vi "DriveControl.vi"(5 "RobotDriveDevRef":T1={"DevStatus"={"status"=FALSE, "code"=0, "source"=""}, "Motors[]"=[], "Square Inputs"=FALSE, "Max Output"=1.0, "Isochronous"=FALSE}, 7 "Xvalue of Target":dbl, 8 "Right axis value":dbl, 9 "Left axis value":dbl, 10 "Lower Bound":dbl, 11 "Upper Bound":dbl) -> (1 "Set Right Speed":dbl, 2 "Set Left Speed":dbl, 3 "RobotDriveDevRef":T1={"DevStatus"={"status"=FALSE, "code"=0, "source"=""}, "Motors[]"=[], "Square Inputs"=FALSE, "Max Output"=1.0, "Isochronous"=FALSE})   [LabVIEW 2011]
uses:
  <vilib>/Rock Robotics/WPI/RobotDrive/WPI_RobotDriveDevRef.ctl
  <vilib>/Rock Robotics/WPI/MotorControl/WPI_MotorControlDeviceRef.ctl
  <vilib>/Rock Robotics/SystemInterfaces/Typedef/FPGA_TypedefDigitalModule.ctl
  <vilib>/Rock Robotics/SystemInterfaces/DIO/FPGA_DIOPWMChannel.ctl
  <vilib>/Rock Robotics/WPI/PWM/WPI_PWMDeadband.ctl
  <vilib>/Rock Robotics/WPI/CAN/Jaguar/SubVIs/WPI_CANJaguar_ControlMode.ctl
  <vilib>/Rock Robotics/WPI/PWM/WPI_PWMTransform_ConPane.ctl
  System Set Points and States.vi
panel:
  in  "Joystick value":dbl
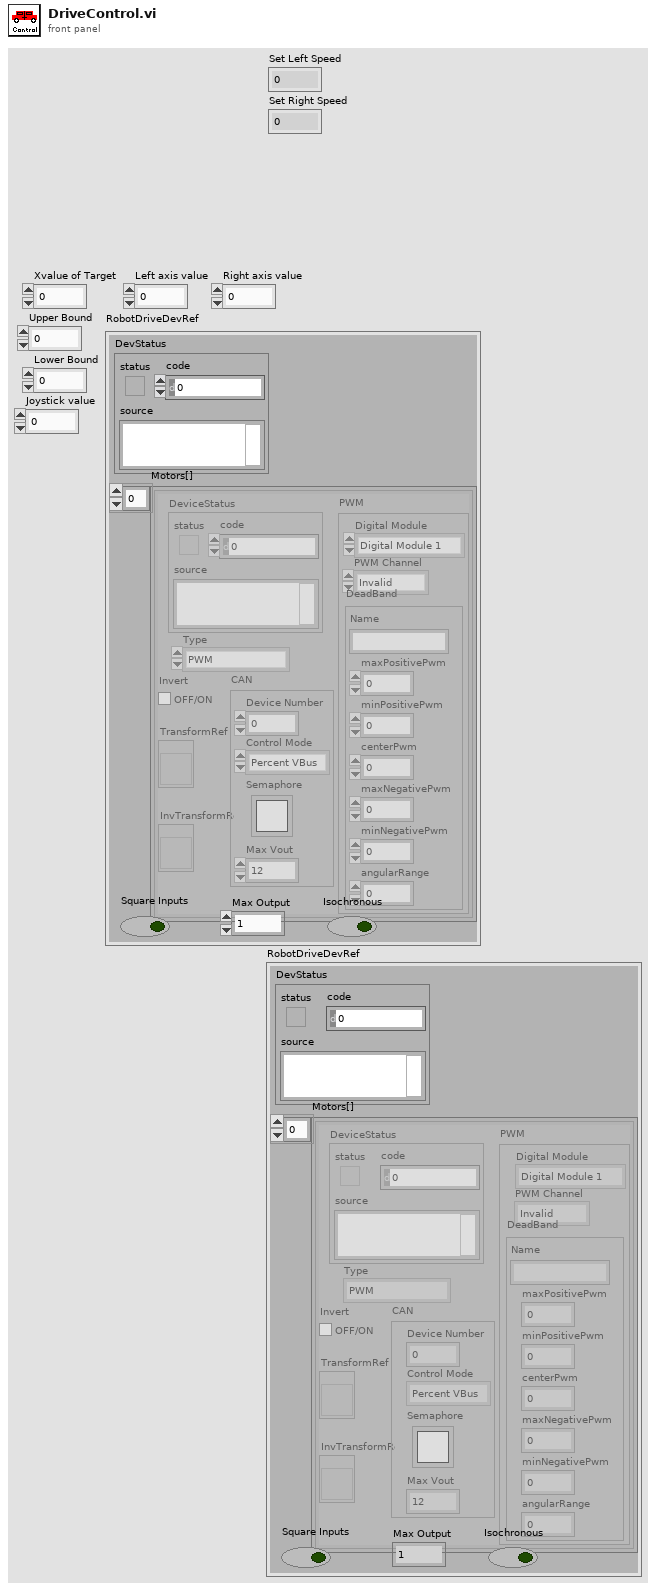
[diagram p1: front panel]
types:
  T1 = typedef "WPI_RobotDriveDevRef.ctl" = cluster{"DevStatus":errorcluster, "Motors[]":T2[], "Square Inputs":bool, "Max Output":dbl, "Isochronous":bool}
  T2 = typedef "WPI_MotorControlDeviceRef.ctl" = cluster{"DeviceStatus":errorcluster, "Type":enum16{"PWM", "CAN"}, "PWM":cluster{"Digital Module":T3, "PWM Channel":T4, "DeadBand":T5}, "CAN":cluster{"Device Number":u8, "Control Mode":T6, "Semaphore":T7, "Max Vout":dbl}, "Invert":bool, "TransformRef":T8, "InvTransformRef":T8}
  T3 = typedef "FPGA_TypedefDigitalModule.ctl" = enum16{"Digital Module 1", "Digital Module 2"}
  T4 = typedef "FPGA_DIOPWMChannel.ctl" = enum8{"PWM 1", "PWM 2", "PWM 3", "PWM 4", "PWM 5", "PWM 6", "PWM 7", "PWM 8", "PWM 9", "PWM 10", "Invalid"}
  T5 = typedef "WPI_PWMDeadband.ctl" = cluster{"Name":string, "maxPositivePwm":i32, "minPositivePwm":i32, "centerPwm":i32, "maxNegativePwm":i32, "minNegativePwm":i32, "angularRange":u16}
  T6 = typedef "WPI_CANJaguar_ControlMode.ctl" = enum8{"Percent VBus", "Current", "Speed", "Position", "Voltage"}
  T7 = typedef "Semaphore RefNum" = refnum<k1>
  T8 = typedef "WPI_PWMTransform_ConPane.ctl" = refnum<vi>
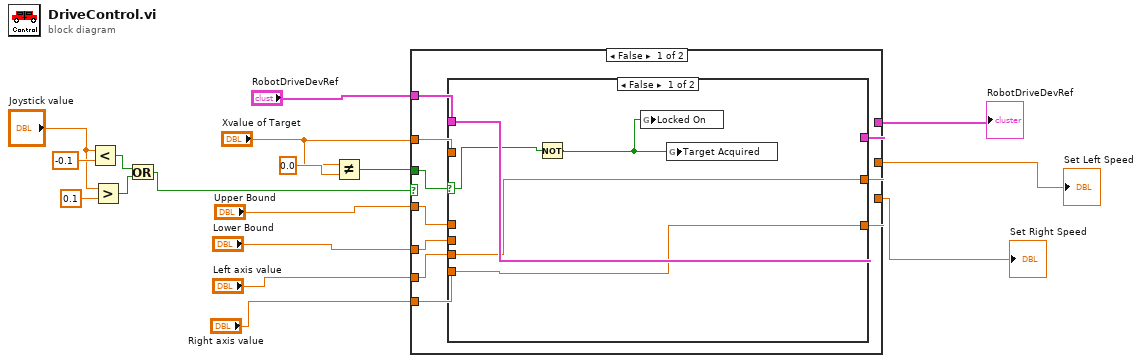
[diagram p0: block diagram]
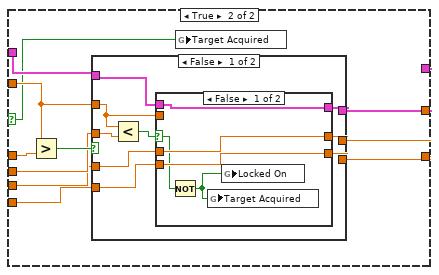
[diagram p2: hidden frame]
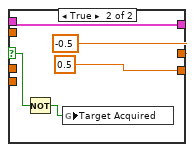
[diagram p3: hidden frame]
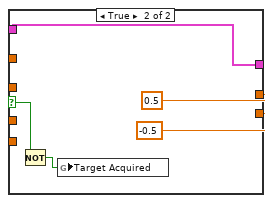
[diagram p4: hidden frame]
diagram:
  n1 = Less?(x="Joystick value", y=-0.1) -> (x < y?=w7:bool)
  n2 = Greater?(x="Joystick value", y=0.1) -> (0:w6:bool)
  n3 = Or(x=w7, y=w6) -> (x .or. y?=w5:bool)
  n4 = Not Equal?(x="Xvalue of Target", y=0.0) -> (x != y?=w1:bool)
  n5 = case shown="False" w5 {
    tunnel: w1 -> [w27 _]
    tunnel: "Xvalue of Target" -> [w26 _]
    tunnel: "Upper Bound" -> [w25 _]
    tunnel: "Lower Bound" -> [w24 _]
    tunnel: "RobotDriveDevRef" -> [w23 w70]
    tunnel: "Left axis value" -> [w22 w69]
    tunnel: "Right axis value" -> [w21 w68]
    tunnel: [w20 w70] -> w4
    tunnel: [w19 w69] -> w3
    tunnel: [w18 w68] -> w2
    frame False {
      n6 = case shown="False" w27 {
        selector: w27 -> [w29 w33]
        tunnel: w26 -> [_ w41]
        tunnel: w25 -> [_ w43]
        tunnel: w24 -> [_ w40]
        tunnel: w23 -> [w32 w39]
        tunnel: w22 -> [w31 w38]
        tunnel: w21 -> [w30 w37]
        tunnel: [w32 w36] -> w20
        tunnel: [w31 w35] -> w19
        tunnel: [w30 w34] -> w18
        frame False {
          n7 = Not(x=w29) -> (.not. x?=w28:bool)
          n8 = global write "System Set Points and States.vi" "Locked On"(w28) -> ()
          n9 = global write "System Set Points and States.vi" "Target Acquired"(w28) -> ()
        }
        frame True {
          n10 = Greater?(x=w41, y=w43) -> (0:w42:bool)
          n11 = case shown="False" w42 {
            selector: w42 -> [_ w63]
            tunnel: w41 -> [w47 _]
            tunnel: w40 -> [w51 _]
            tunnel: w39 -> [w50 w67]
            tunnel: w38 -> [w49 _]
            tunnel: w37 -> [w48 _]
            tunnel: [w46 w67] -> w36
            tunnel: [w45 0.5 ("Left axis value")] -> w35
            tunnel: [w44 -0.5 ("Right axis value")] -> w34
            frame False {
              n12 = Less?(x=w47, y=w51) -> (x < y?=w52:bool)
              n13 = case shown="False" w52 {
                selector: w52 -> [w54 w58]
                tunnel: w50 -> [w57 w62]
                tunnel: w49 -> [w56 _]
                tunnel: w48 -> [w55 _]
                tunnel: w47 -> [_ _]
                tunnel: [w57 w62] -> w46
                tunnel: [w56 -0.5 ("Left axis value")] -> w45
                tunnel: [w55 0.5 ("Right axis value")] -> w44
                frame False {
                  n14 = Not(x=w54) -> (.not. x?=w53:bool)
                  n15 = global write "System Set Points and States.vi" "Target Acquired"(w53) -> ()
                  n16 = global write "System Set Points and States.vi" "Locked On"(w53) -> ()
                }
                frame True {
                  n17 = Not(x=w58) -> (.not. x?=w59:bool)
                  n18 = global write "System Set Points and States.vi" "Target Acquired"(w59) -> ()
                }
              }
            }
            frame True {
              n19 = Not(x=w63) -> (.not. x?=w64:bool)
              n20 = global write "System Set Points and States.vi" "Target Acquired"(w64) -> ()
            }
          }
          n21 = global write "System Set Points and States.vi" "Target Acquired"(w33) -> ()
        }
      }
    }
    frame True {
    }
  }
  "RobotDriveDevRef" <- w4
  "Set Left Speed" <- w3
  "Set Right Speed" <- w2
